vi "Stop.vi"(8 "error in":errorcluster, 11 "Virtual Voltmeter in":refnum<class "Virtual Voltmeter.lvclass">) -> (0 "error out":errorcluster, 3 "Virtual Voltmeter out":refnum<class "Virtual Voltmeter.lvclass">)   [LabVIEW 2023, in "Voltmeter.lvlib" / "Virtual Voltmeter.lvlib" / "Virtual Voltmeter.lvclass"]
uses:
  Virtual Voltmeter.lvclass
  Virtual Voltmeter.lvclass/Virtual Voltmeter.ctl
  Interfaces/IRead Voltage Multichannel/IRead Voltage from Channel.lvclass
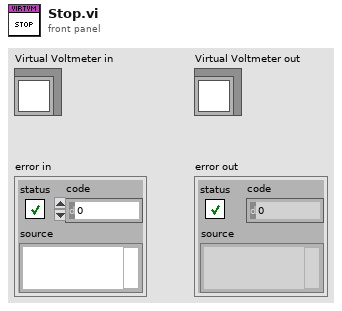
[diagram p1: front panel]
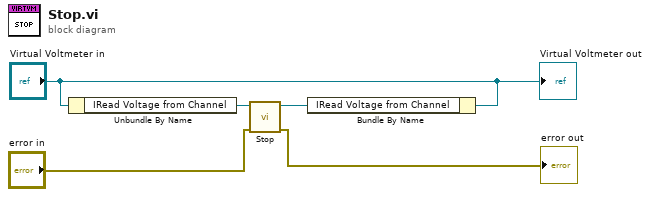
[diagram p0: block diagram]
diagram:
  n1 = Unbundle By Name("Virtual Voltmeter in") -> ("IRead Voltage from Channel"=w5:refnum<class "IRead Voltage from Channel.lvclass">)
  n2 = call-dynamic "Stop.vi"("error in"="error in", "IRead Voltage in"=w5) -> ("error out"=→"error out":errorcluster, "IRead Voltage out"=w2:refnum<class "IRead Voltage from Channel.lvclass">)  [unwired: 8 in]
  n3 = Bundle By Name(cluster="Virtual Voltmeter in", "IRead Voltage from Channel"=w2) -> ()  [unwired: 1 out]
  "Virtual Voltmeter out" <- "Virtual Voltmeter in"
